vi "Choreo_Trajectory_New_Empty.vi"() -> (3 "ChoreoTrajectory":T1)   [LabVIEW 2019, in "ChoreoLib.lvlib"]
doc: "Inputs: \n\nOutputs:"
uses:
  ChoreoLib.lvlib
  TypeDef/ChoreoTrajectory.ctl
  TypeDef/ChoreoTrajectoryState.ctl
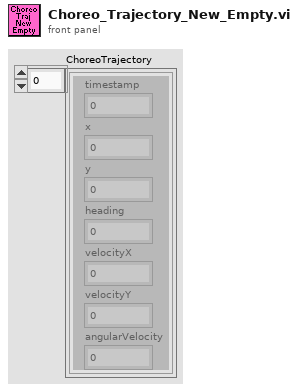
[diagram p1: front panel]
types:
  T1 = typedef "ChoreoLib.lvlib/ChoreoTrajectory.ctl" = T2[]
  T2 = typedef "ChoreoLib.lvlib/ChoreoTrajectoryState.ctl" = cluster{"timestamp":dbl, "x":dbl, "y":dbl, "heading":dbl, "velocityX":dbl, "velocityY":dbl, "angularVelocity":dbl}
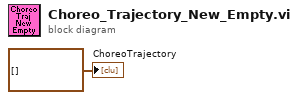
[diagram p0: block diagram]
diagram:
  "ChoreoTrajectory" <- T1 [] ("ChoreoTrajectory")
